vi "Simple_Camram_Example_IMAQ.vi"() -> ()   [LabVIEW 2019]
uses:
  camera/Camera.lvclass
panel:
  out "rawImage":u16[][](array[numeric])
  out "Image":T1(plugin-control)
  in  "data_format":T2(ring)=enum."Mono16"
  in  "Image Index":u32 max=2
  out "Recorded Images":u32
  in  "Quit":bool
  in  "roiY1":u64=2 min=2 max=2016 step=1
  in  "roiX1":u64=2 min=2 max=2016 step=1
  in  "roiY0":u64=1 min=1 max=2015 step=1
  in  "roiX0":u64=1 min=1 max=2015 step=1
  out "Image Height":u16
  out "Image Width":u16
  in  "segment":u16=3 caption="Segment" min=1 max=4
  out "Error":errorcluster {"code" format="%x"}
  # "This example shows for cameras with internal memory how to setup and record into a segment and show the images after record finished\nIt is a good starting point for writing own applications.\nBut it will not be fail save, i.e. doesnt react on errors, just handles them forward to the end\n\nUsage:\nSelect the segment you want to record into before you start the program.\nOnce started, the camera class will be initialized and images will be recorded automatically.\nWhen acquisition has finished you can address the images and set a certain roi \nTo finish the program click on quit application, this will force fan exit of the camera class"
  # "pco.labview"
  # "Camera Setup"
  # "Recording Control"
  # "Parameters for image readout"
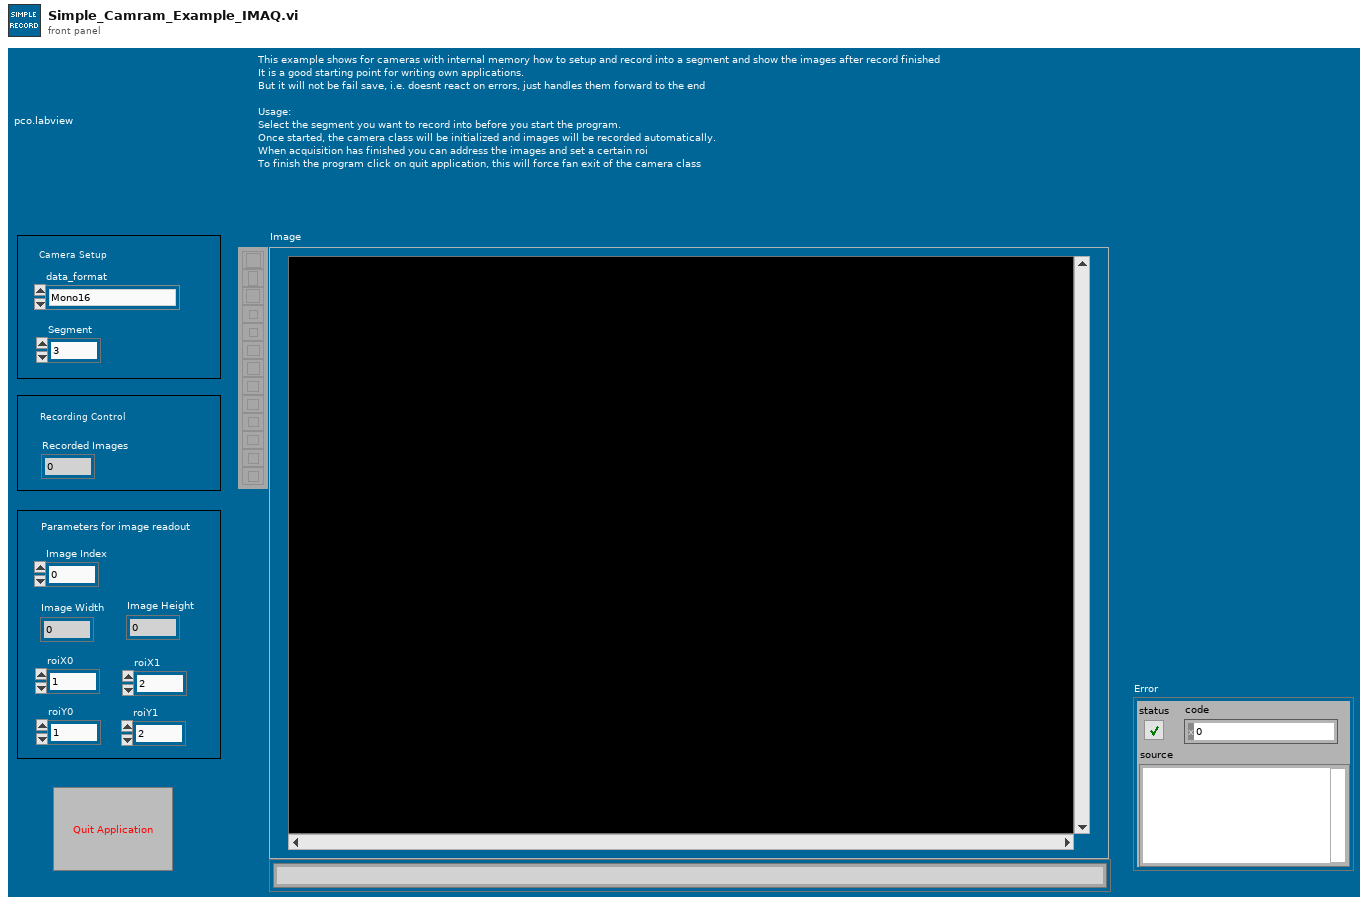
[diagram p1: front panel]
types:
  T1 = typedef "IMAQ Image.ctl" = refnum<image>
  T2 = enum16{"Undefined", "Mono8", "Mono16", "BGRA8", "RGBA8", "BGRA16", "RGBA16", "CompressedMono8"}
  T3 = enum8{"Enabled", "Disabled", "Disabled and Grayed Out"}
  T4 = enum16{"sequence", "sequence non blocking", "ring buffer", "fifo", "tif", "multitif", "pcoraw", "b16", "dicom", "multidicom", "camram_ring", "camram_segment"}
  T5 = cluster{"serial":u32, "type":u16, "sub_type":u16, "interface_type":u16, "bit_resolution":u16, "min_exposure_time_s":dbl, "max_exposure_time_s":dbl, "min_exposure_step_s":dbl, "min_delay_time_s":dbl, "max_delay_time_s":dbl, "min_delay_step_s":dbl, "min_width":u64, "min_height":u64, "max_width":u64, "max_height":u64, "roi_step_horz":u64, "roi_step_vert":u64, "roi_symmetric_horz":bool, "roi_symmetric_vert":bool, "has_timestamp_mode":bool, "has_timestamp_mode_ascii_only":bool, "pixelrate_vec":u32[], "conversion_factor_vec":sgl[], "has_trigger_mode_extexpctrl":bool, "has_acquire_mode":bool, "has_ext_acquire_mode":bool, "has_metadata_mode":bool, "has_ram":bool, "binning_horz_vec":u16[], "binning_vert_vec":u16[], "has_average_binning":bool, "pixel_format_vec":u32[]}
  T6 = typedef "Image Type" = u32
  T7 = typedef "Camera.lvclass/binning.ctl" = cluster{"vert":u16, "horz":u16, "mode":u16}
  T8 = cluster{"exposure_time_s":dbl, "delay_time_s":dbl, "roi":cluster{"x0":u64, "y0":u64, "x1":u64, "y1":u64}, "timestamp_mode":u16, "pixelrate":u32, "conversion_factor":sgl, "trigger_mode":u16, "acquire_mode":u16, "acquire_sequence_number":u32, "metadata_mode":u16, "noisefilter_mode":u16, "pixel_format":u32, "binning":T7, "auto_exposure":cluster{"region":u16, "min_exposure_s":dbl, "max_exposure_s":dbl}}
  T9 = cluster{"Plane 4 (alpha)":u16, "Plane 1 (Red)":u16, "Plane 2 (Green)":u16, "Plane 3 (Blue)":u16}[][]
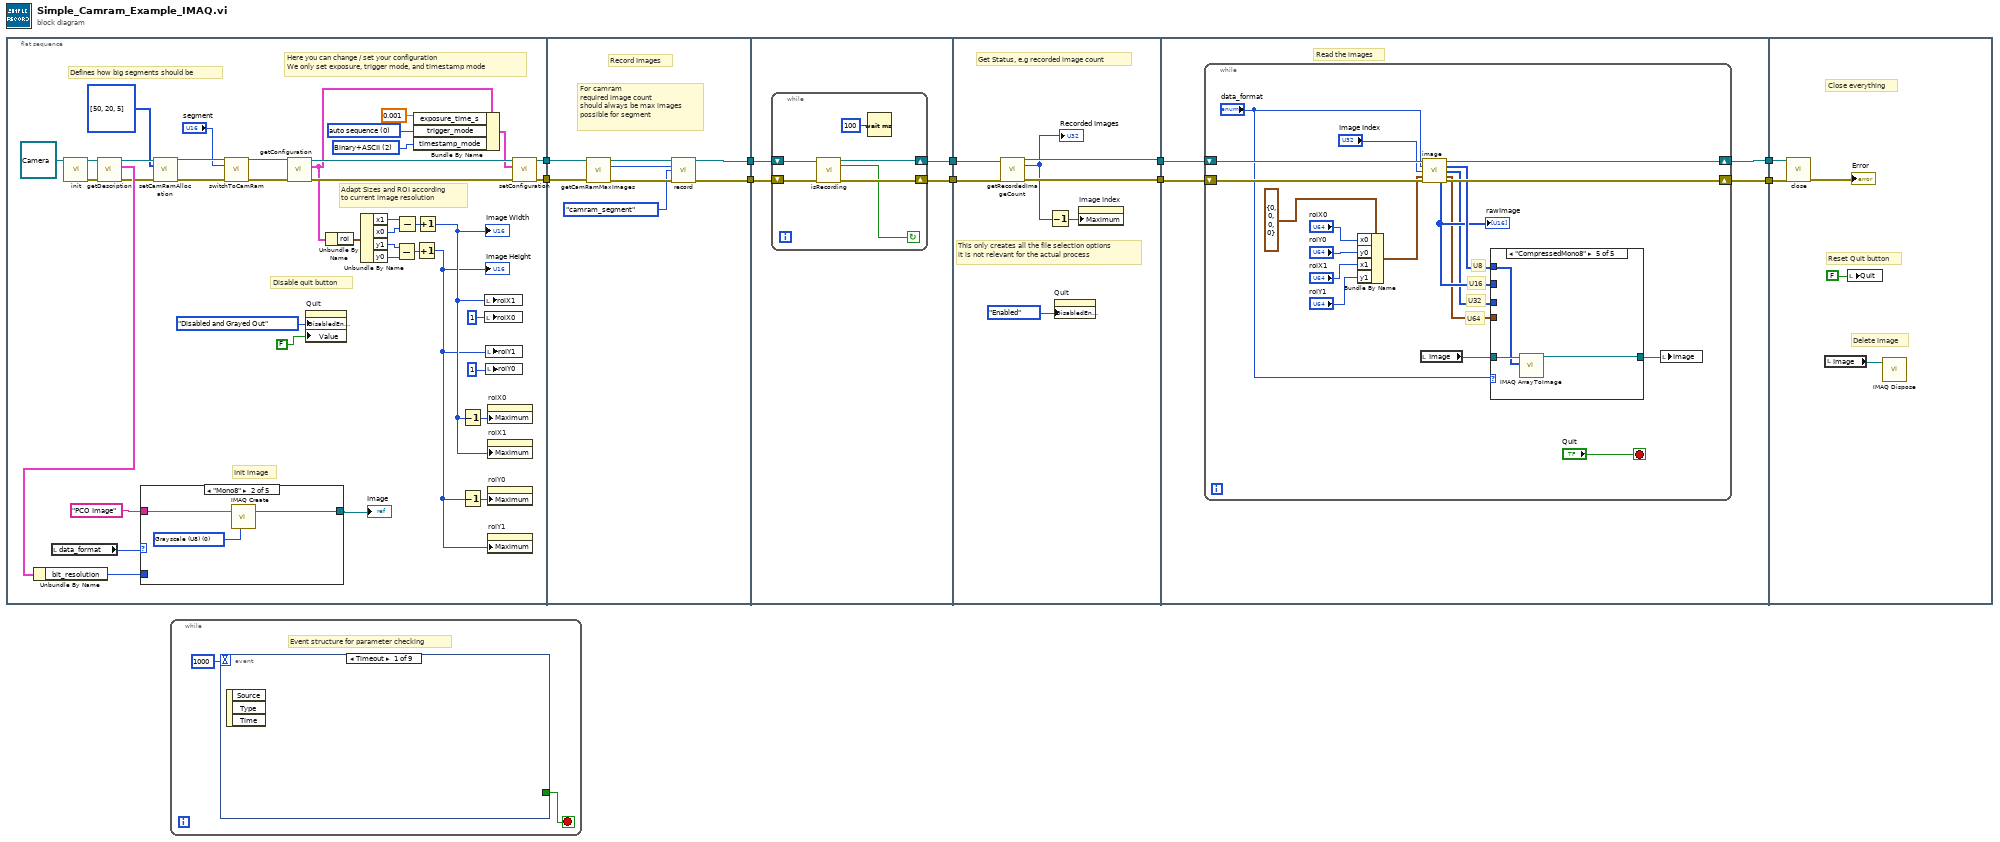
[diagram p0: block diagram]
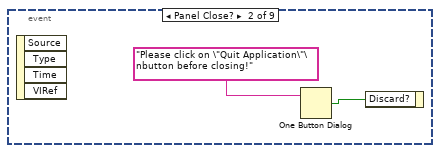
[diagram p2: hidden frame]
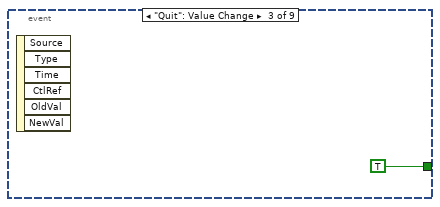
[diagram p3: hidden frame]
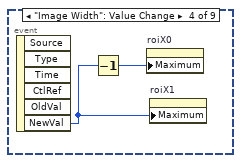
[diagram p4: hidden frame]
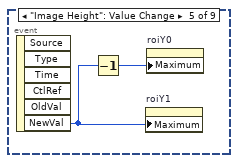
[diagram p5: hidden frame]
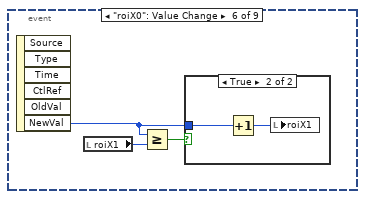
[diagram p6: hidden frame]
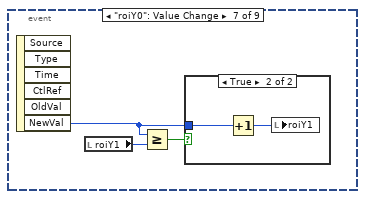
[diagram p8: hidden frame]
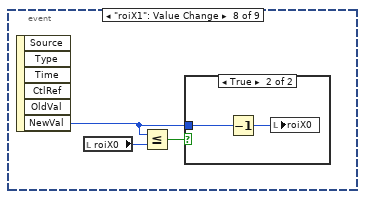
[diagram p10: hidden frame]
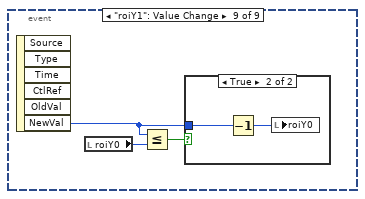
[diagram p12: hidden frame]
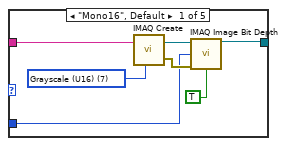
[diagram p14: hidden frame]
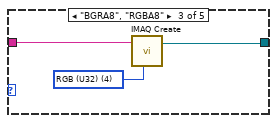
[diagram p15: hidden frame]
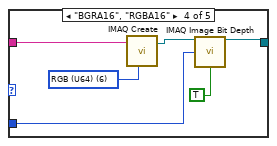
[diagram p16: hidden frame]
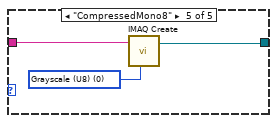
[diagram p17: hidden frame]
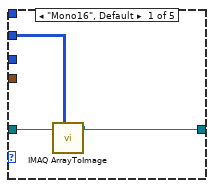
[diagram p18: hidden frame]
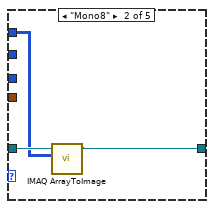
[diagram p19: hidden frame]
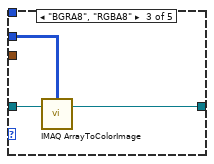
[diagram p20: hidden frame]
diagram:
  n1 = flat-sequence {
    tunnel: [w45] -> w10
    tunnel: [w44] -> w9
    tunnel: w10 -> [w77]
    tunnel: w9 -> [w78]
    tunnel: [w80] -> w4
    tunnel: [w79] -> w2
    tunnel: w4 -> [w84]
    tunnel: [w81] -> w3
    tunnel: w2 -> [w83]
    tunnel: [w82] -> w1
    tunnel: w3 -> [w97]
    tunnel: w1 -> [w96]
    tunnel: [w95] -> w8
    tunnel: [w94] -> w7
    tunnel: w8 -> [w100]
    tunnel: w7 -> [w101]
    tunnel: [w99] -> w6
    tunnel: [w98] -> w5
    tunnel: w6 -> [w138]
    tunnel: w5 -> [w137]
    frame #0 {
      w29 = u16 2 items=["OFF", "Binary", "Binary+ASCII", "ASCII"] ("TimestampMode")
      w49 = u16 0 items=["auto sequence"=0, "software trigger"=1, "external exposure start & software trigger"=2, "external exposure control"=3, "external synchronized"=4, "fast external exposure control"=5, "external CDS control"=6, "slow external exposure control"=7, "external synchronized HDSDI"=258] ("TriggerMode")
      # "Here you can change / set your configuration\nWe only set exposure, trigger mode, and timestamp mode"
      # "Defines how big segments should be"
      # "Init image"
      # "Adapt Sizes and ROI according\nto current image resolution"
      # "Disable quit button"
      n2 = local read "data_format"() -> (w26:T2)
      n3 = call-dynamic "init.vi"("Camera in"=refnum<class "Camera.lvclass"> refnum ("PCOCamera in")) -> ("Camera out"=w22:refnum<class "Camera.lvclass">, "error out"=w23:errorcluster)  [unwired: 8 in]
      n4 = call-dynamic "getDescription.vi"("error in (no error)"=w23, "Camera in"=w22) -> ("error out"=w18:errorcluster, "description"=w21:T5, "Camera out"=w17:refnum<class "Camera.lvclass">)  [unwired: 7 in]
      n5 = Unbundle By Name(w21) -> ("bit_resolution"=w20:u16)
      n6 = case shown="\"Mono8\"" w26 {
        tunnel: "PCO Image" ("Image Name") -> [w56 w60 w62 w68 w71]
        tunnel: [w52 w58 w61 w65 w70] -> w25
        tunnel: w20 -> [w51 _ _ w64 _]
        frame "Mono16", Default {
          w57 = T6 7 items=["Grayscale (U8)", "Grayscale (I16)", "Grayscale (SGL)", "Complex (CSG)", "RGB (U32)", "HSL (U32)", "RGB (U64)", "Grayscale (U16)"] ("Image Type")
          n7 = call "IMAQ Create"("Image Name"=w56, "Image Type"=w57) -> ("New Image"=w54:T1, "error out"=w53:errorcluster)  [unwired: 3 in]
          n8 = call "IMAQ Image Bit Depth"("Image"=w54, "Bit Depth (0)"=w51, "error in (no error)"=w53, "Get/Set Bit Depth? (Set)"=TRUE) -> ("Image Out"=w52:T1)  [unwired: 9 in, 2 out]
        }
        frame "Mono8" {
          w59 = T6 0 items=["Grayscale (U8)", "Grayscale (I16)", "Grayscale (SGL)", "Complex (CSG)", "RGB (U32)", "HSL (U32)", "RGB (U64)", "Grayscale (U16)"] ("Image Type")
          n9 = call "IMAQ Create"("Image Name"=w60, "Image Type"=w59) -> ("New Image"=w58:T1)  [unwired: 3 in, 1 out]
        }
        frame "BGRA8", "RGBA8" {
          w63 = T6 4 items=["Grayscale (U8)", "Grayscale (I16)", "Grayscale (SGL)", "Complex (CSG)", "RGB (U32)", "HSL (U32)", "RGB (U64)", "Grayscale (U16)"] ("Image Type")
          n10 = call "IMAQ Create"("Image Name"=w62, "Image Type"=w63) -> ("New Image"=w61:T1)  [unwired: 3 in, 1 out]
        }
        frame "BGRA16", "RGBA16" {
          w69 = T6 6 items=["Grayscale (U8)", "Grayscale (I16)", "Grayscale (SGL)", "Complex (CSG)", "RGB (U32)", "HSL (U32)", "RGB (U64)", "Grayscale (U16)"] ("Image Type")
          n11 = call "IMAQ Create"("Image Name"=w68, "Image Type"=w69) -> ("New Image"=w66:T1)  [unwired: 3 in, 1 out]
          n12 = call "IMAQ Image Bit Depth"("Image"=w66, "Bit Depth (0)"=w64, "Get/Set Bit Depth? (Set)"=TRUE) -> ("Image Out"=w65:T1)  [unwired: 10 in, 2 out]
        }
        frame "CompressedMono8" {
          w72 = T6 0 items=["Grayscale (U8)", "Grayscale (I16)", "Grayscale (SGL)", "Complex (CSG)", "RGB (U32)", "HSL (U32)", "RGB (U64)", "Grayscale (U16)"] ("Image Type")
          n13 = call "IMAQ Create"("Image Name"=w71, "Image Type"=w72) -> ("New Image"=w70:T1)  [unwired: 3 in, 1 out]
        }
      }
      "Image" <- w25
      n14 = call-dynamic "setCamRamAllocation.vi"("Camera in"=w17, "percents"=u32[] [50, 20, 5], "error in (no error)"=w18) -> ("Camera out"=w16:refnum<class "Camera.lvclass">, "error out"=w19:errorcluster)  [unwired: 11 in]
      n15 = call-dynamic "switchToCamRam.vi"("Camera in"=w16, "segment"="segment", "error in (no error)"=w19) -> ("Camera out"=w15:refnum<class "Camera.lvclass">, "error out"=w14:errorcluster)  [unwired: 11 in]
      n16 = call-dynamic "getConfiguration.vi"("error in (no error)"=w14, "Camera in"=w15) -> ("error out"=w47:errorcluster, "configuration"=w39:T8, "Camera out"=w48:refnum<class "Camera.lvclass">)  [unwired: 7 in]
      n17 = property on="Quit" class="Bool (strict)"("DisabledEnum"=T3."Disabled and Grayed Out" ("Disabled"), "Value"=FALSE ("Stop")) -> ()  [unwired: 2 in, 2 out]
      n18 = Unbundle By Name(w39) -> ("roi"=w38:cluster{"x0":u64, "y0":u64, "x1":u64, "y1":u64})
      n19 = Unbundle By Name(w38) -> ("x1"=w36:u64, "x0"=w37:u64, "y1"=w34:u64, "y0"=w35:u64)
      n20 = Subtract(x=w34, y=w35) -> (x-y=w32:u64)
      n21 = Subtract(x=w36, y=w37) -> (x-y=w33:u64)
      n22 = Bundle By Name(cluster=w39, "exposure_time_s"=0.001, "trigger_mode"=w49, "timestamp_mode"=w29) -> (w46:T8)
      n23 = Increment(x=w32) -> (x+1=w30:u64)
      "Image Height" <- w30
      n24 = Increment(x=w33) -> (x+1=w31:u64)
      "Image Width" <- w31
      n25 = Decrement(x=w31) -> (x-1=w41:u64)
      n26 = Decrement(x=w30) -> (x-1=w40:u64)
      n27 = local write "roiX1"(w31) -> ()
      n28 = local write "roiX0"(u16 1 ("roiY0")) -> ()
      n29 = local write "roiY1"(w30) -> ()
      n30 = local write "roiY0"(u16 1 ("roiY0")) -> ()
      n31 = property on="roiX0" class="DigNum (strict)"("Maximum"=w41) -> ()  [unwired: 2 in, 2 out]
      n32 = property on="roiX1" class="DigNum (strict)"("Maximum"=w31) -> ()  [unwired: 2 in, 2 out]
      n33 = property on="roiY0" class="DigNum (strict)"("Maximum"=w40) -> ()  [unwired: 2 in, 2 out]
      n34 = property on="roiY1" class="DigNum (strict)"("Maximum"=w30) -> ()  [unwired: 2 in, 2 out]
      n35 = call-dynamic "setConfiguration.vi"("error in (no error)"=w47, "configuration"=w46, "Camera in"=w48) -> ("error out"=w44:errorcluster, "Camera out"=w45:refnum<class "Camera.lvclass">)  [unwired: 7 in]
    }
    frame #1 {
      # "For camram\nrequired image count \nshould always be max images\npossible for segment"
      # "Record Images"
      n36 = call-dynamic "getCamRamMaxImages.vi"("Camera in"=w77, "error in (no error)"=w78) -> ("Camera out"=w74:refnum<class "Camera.lvclass">, "max_images"=w75:u32, "error out"=w76:errorcluster)  [unwired: 11 in]
      n37 = call-dynamic "record.vi"("Camera in"=w74, "num_images"=w75, "record_mode"=T4."camram_segment", "error in (no error)"=w76) -> ("Camera out"=w80:refnum<class "Camera.lvclass">, "error out"=w79:errorcluster)  [unwired: 10 in]
    }
    frame #2 {
      n38 = while {
        shift-right: [w88] -> w82
        shift-left: w83 -> [w89]
        shift-right: [w87] -> w81
        shift-left: w84 -> [w90]
        stop <- w85 continue-if-true
        n39 = call-dynamic "isRecording.vi"("Camera in"=w90, "error in (no error)"=w89) -> ("Camera out"=w87:refnum<class "Camera.lvclass">, "recording"=w85:bool, "error out"=w88:errorcluster)  [unwired: 11 in]
        n40 = Wait (ms)(milliseconds to wait=u32 100) -> ()  [unwired: 1 out]
      }
    }
    frame #3 {
      # "This only creates all the file selection options\nit is not relevant for the actual process"
      # "Get Status, e.g recorded image count"
      n41 = call-dynamic "getRecordedImageCount.vi"("Camera in"=w97, "error in (no error)"=w96) -> ("Camera out"=w95:refnum<class "Camera.lvclass">, "recorded_image_count"=w91:u32, "error out"=w94:errorcluster)  [unwired: 11 in]
      "Recorded Images" <- w91
      n42 = Decrement(x=w91) -> (x-1=w92:u32)
      n43 = property on="Quit" class="Bool (strict)"("DisabledEnum"=T3."Enabled" ("Disabled")) -> ()  [unwired: 2 in, 2 out]
      n44 = property on="Image Index" class="DigNum (strict)"("Maximum"=w92) -> ()  [unwired: 2 in, 2 out]
    }
    frame #4 {
      # "Read the images"
      n45 = while {
        shift-right: [w118] -> w99
        shift-left: w100 -> [w120]
        shift-right: [w113] -> w98
        shift-left: w101 -> [w119]
        stop <- "Quit" stop-if-true
        # "U64"
        # "U32"
        # "U16"
        # "U8"
        n46 = Bundle By Name(cluster=cluster{"x0":u64, "y0":u64, "x1":u64, "y1":u64} {"x0"=0, "y0"=0, "x1"=0, "y1"=0} ("roi"), "x0"="roiX0", "y0"="roiY0", "x1"="roiX1", "y1"="roiY1") -> (w112:cluster{"x0":u64, "y0":u64, "x1":u64, "y1":u64})
        n47 = local read "Image"() -> (w105:T1)
        n48 = call-dynamic "image.vi"("Camera in"=w120, "data_format"="data_format", "image_index"="Image Index", "crop"=w112, "error in (no error)"=w119) -> ("Camera out"=w118:refnum<class "Camera.lvclass">, "image (U8)"=w109:u8[][], "image (U32)"=w107:u32[][], "image (U64)"=w106:T9, "raw_image (U16)"=w108:u16[][], "error out"=w113:errorcluster)  [unwired: 2 in, 3 out]
        "rawImage" <- w108
        n49 = case shown="\"CompressedMono8\"" "data_format" {
          tunnel: w105 -> [w123 w126 w129 w132 w135]
          tunnel: [w121 w124 w128 w130 w134] -> w104
          tunnel: w106 -> [_ _ _ w131 _]
          tunnel: w107 -> [_ _ w127 _ _]
          tunnel: w109 -> [_ w125 _ _ w133]
          tunnel: w108 -> [w122 _ _ _ _]
          frame "Mono16", Default {
            n50 = call "IMAQ ArrayToImage"("Image Pixels (U16)"=w122, "Image"=w123) -> ("Image Out"=w121:T1)  [unwired: 8 in, 1 out]
          }
          frame "Mono8" {
            n51 = call "IMAQ ArrayToImage"("Image Pixels (U8)"=w125, "Image"=w126) -> ("Image Out"=w124:T1)  [unwired: 8 in, 1 out]
          }
          frame "BGRA8", "RGBA8" {
            n52 = call "IMAQ ArrayToColorImage"("Image Pixels (U32)"=w127, "Image"=w129) -> ("Image Out"=w128:T1)  [unwired: 3 in, 1 out]
          }
          frame "BGRA16", "RGBA16" {
            n53 = call "IMAQ ArrayToColorImage"("Image"=w132, "Image Pixels (U64)"=w131) -> ("Image Out"=w130:T1)  [unwired: 3 in, 1 out]
          }
          frame "CompressedMono8" {
            n54 = call "IMAQ ArrayToImage"("Image Pixels (U8)"=w133, "Image"=w135) -> ("Image Out"=w134:T1)  [unwired: 8 in, 1 out]
          }
        }
        n55 = local write "Image"(w104) -> ()
      }
    }
    frame #5 {
      # "Delete image"
      # "Reset Quit button"
      # "Close everything"
      n56 = call-dynamic "close.vi"("error in (no error)"=w137, "Camera in"=w138) -> ("error out"=→"Error":errorcluster)  [unwired: 9 in]
      n57 = local read "Image"() -> (w136:T1)
      n58 = local write "Quit"(FALSE ("Stop")) -> ()
      n59 = call "IMAQ Dispose"("Image"=w136) -> ()  [unwired: 5 in, 1 out]
    }
  }
  n60 = while {
    stop <- w141 stop-if-true
    # "Event structure for parameter checking"
    n61 = event shown="[0] Timeout" {
      selector: _ -> [_ _ _ _ _ _ _ _ _]
      dyn-events: _ -> [_ _ _ _ _ _ _ _ _]
      timeout: 1000 -> [_ _ _ _ _ _ _ _ _]
      tunnel: [_ _ TRUE _ _ _ _ _ _] -> w141
      event Timeout {
        n62 = event-data() -> ()  [unwired: 1 in, 3 out]
      }
      event Panel Close? {
        n63 = event-data() -> ()  [unwired: 1 in, 4 out]
        n64 = One Button Dialog(message="Please click on \"Quit Application\"\nbutton before closing!") -> (true=w143:bool)  [unwired: 1 in]
        n65 = event-data("Discard?"=w143) -> ()  [unwired: 1 in, 1 out]
      }
      event "Quit": Value Change {
        n66 = event-data() -> ()  [unwired: 1 in, 6 out]
      }
      event "Image Width": Value Change {
        n67 = event-data() -> ("NewVal"=w146:u16)  [unwired: 1 in, 5 out]
        n68 = Decrement(x=w146) -> (x-1=w147:u16)
        n69 = property on="roiX0" class="DigNum (strict)"("Maximum"=w147) -> ()  [unwired: 2 in, 2 out]
        n70 = property on="roiX1" class="DigNum (strict)"("Maximum"=w146) -> ()  [unwired: 2 in, 2 out]
      }
      event "Image Height": Value Change {
        n71 = event-data() -> ("NewVal"=w148:u16)  [unwired: 1 in, 5 out]
        n72 = Decrement(x=w148) -> (x-1=w149:u16)
        n73 = property on="roiY1" class="DigNum (strict)"("Maximum"=w148) -> ()  [unwired: 2 in, 2 out]
        n74 = property on="roiY0" class="DigNum (strict)"("Maximum"=w149) -> ()  [unwired: 2 in, 2 out]
      }
      event "roiX0": Value Change {
        n75 = event-data() -> ("NewVal"=w150:u64)  [unwired: 1 in, 5 out]
        n76 = local read "roiX1"() -> (w152:u64)
        n77 = Greater Or Equal?(x=w150, y=w152) -> (x >= y?=w151:bool)
        n78 = case shown="True" w151 {
          tunnel: w150 -> [_ w154]
          frame False {
          }
          frame True {
            n79 = Increment(x=w154) -> (x+1=w153:u64)
            n80 = local write "roiX1"(w153) -> ()
          }
        }
      }
      event "roiY0": Value Change {
        n81 = event-data() -> ("NewVal"=w155:u64)  [unwired: 1 in, 5 out]
        n82 = local read "roiY1"() -> (w157:u64)
        n83 = Greater Or Equal?(x=w155, y=w157) -> (x >= y?=w156:bool)
        n84 = case shown="True" w156 {
          tunnel: w155 -> [_ w159]
          frame False {
          }
          frame True {
            n85 = Increment(x=w159) -> (x+1=w158:u64)
            n86 = local write "roiY1"(w158) -> ()
          }
        }
      }
      event "roiX1": Value Change {
        n87 = event-data() -> ("NewVal"=w160:u64)  [unwired: 1 in, 5 out]
        n88 = local read "roiX0"() -> (w162:u64)
        n89 = Less Or Equal?(x=w160, y=w162) -> (x <= y?=w161:bool)
        n90 = case shown="True" w161 {
          tunnel: w160 -> [_ w164]
          frame False {
          }
          frame True {
            n91 = Decrement(x=w164) -> (x-1=w163:u64)
            n92 = local write "roiX0"(w163) -> ()
          }
        }
      }
      event "roiY1": Value Change {
        n93 = event-data() -> ("NewVal"=w165:u64)  [unwired: 1 in, 5 out]
        n94 = local read "roiY0"() -> (w167:u64)
        n95 = Less Or Equal?(x=w165, y=w167) -> (x <= y?=w166:bool)
        n96 = case shown="True" w166 {
          tunnel: w165 -> [_ w169]
          frame False {
          }
          frame True {
            n97 = Decrement(x=w169) -> (x-1=w168:u64)
            n98 = local write "roiY0"(w168) -> ()
          }
        }
      }
    }
  }
